vi "niScope Multi Read Cluster.vi"(7 "timeout":dbl=5.0 format="%.2f", 8 "error in":errorcluster, 9 "numSamples":i32=-1, 10 "channels":string="0", 11 "instrument handle":refnum<k15>) -> (0 "error out":errorcluster, 1 "waveform":T2(array[cluster]) {"wfm" format="%.2f"; "xIncrement" format="%.2f"; "relativeInitialX" format="%.2f"}, 2 "wfm info":T1(array[cluster]) {"reserved2" format="%.2f"; "reserved1" format="%.2f"; "offset" format="%^.3e"; "gain" format="%^.3e"; "xIncrement" format="%^.3e"; "relativeInitialX" format="%^.3e"; "absoluteInitialX" format="%^.3e"}, 3 "instrument handle out":refnum<k15>)   [LabVIEW 2013]
doc: "Initiates an acquisition, waits for it to complete, and retrieves the data for multiple channels and records."
uses:
  niScope_32.dll
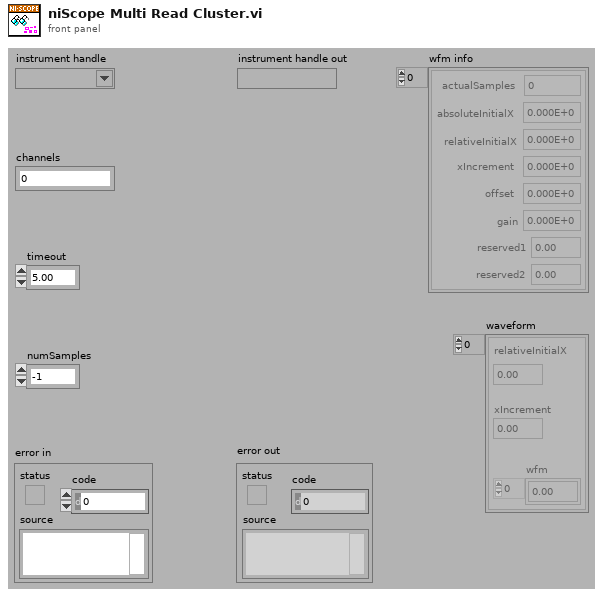
[diagram p1: front panel]
types:
  T1 = cluster{"actualSamples":i32, "absoluteInitialX":dbl, "relativeInitialX":dbl, "xIncrement":dbl, "offset":dbl, "gain":dbl, "reserved1":dbl, "reserved2":dbl}[]
  T2 = cluster{"relativeInitialX":dbl, "xIncrement":dbl, "wfm":dbl[]}[]
  T3 = cluster{"relativeInitialX":dbl, "xIncrement":dbl, "wfm":dbl[]}
  T4 = cluster{"actualSamples":i32, "absoluteInitialX":dbl, "relativeInitialX":dbl, "xIncrement":dbl, "offset":dbl, "gain":dbl, "reserved1":dbl, "reserved2":dbl}
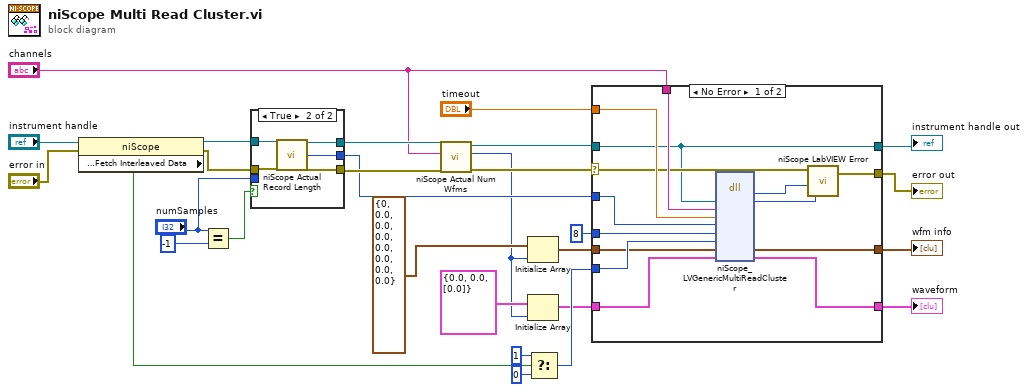
[diagram p0: block diagram]
diagram:
  n1 = property class="niScope"(reference="instrument handle", error in="error in") -> (reference out=w10:refnum<k15>, error out=w20:errorcluster, "Device Specific:IF Digitizer (5620 and 5621):Advanced:Fetch Interleaved Data"=w21:bool)
  n2 = Equal?(x="numSamples", y=-1) -> (x = y?=w27:bool)
  n3 = case shown="True" w27 {
    tunnel: [w29 w36] -> w24
    tunnel: [w30 w35] -> w25
    tunnel: "numSamples" -> [w31 _]
    tunnel: [w31 w34] -> w15
    tunnel: w10 -> [w30 w33]
    tunnel: w20 -> [w29 w32]
    frame False {
    }
    frame True {
      n4 = call <instrlib>:"niScope Actual Record Length.vi"("instrument handle"=w33, "error in"=w32) -> ("instrument handle out"=w35:refnum<k15>, "actual record length"=w34:i32, "error out"=w36:errorcluster)  [unwired: 11 in]
    }
  }
  n5 = call <instrlib>:"niScope Actual Num Wfms.vi"("error in"=w24, "channels"="channels", "instrument handle"=w25) -> ("error out"=w14:errorcluster, "actual num wfms"=w3:i32, "instrument handle out"=w13:refnum<k15>)  [unwired: 6 in]
  n6 = Initialize Array(T4 {"actualSamples"=0, "absoluteInitialX"=0.0, "relativeInitialX"=0.0, "xIncrement"=0.0, "offset"=0.0, "gain"=0.0, "reserved1"=0.0, "reserved2"=0.0} ("wfm info"), w3) -> (w2:T1)
  n7 = Initialize Array(T3 {"relativeInitialX"=0.0, "xIncrement"=0.0, "wfm"=[0.0]}, w3) -> (w1:T2)
  n8 = Select(t=1, s=w21, f=0) -> (s? t:f=w16:i32)
  n9 = case shown="No Error" w14 {
    selector: w14 -> [w38 w53]
    tunnel: [w48 w53] -> w6
    tunnel: w13 -> [w37 w54]
    tunnel: [w37 w54] -> w9
    tunnel: w15 -> [w39 _]
    tunnel: [w45 w51] -> w8
    tunnel: w16 -> [w44 _]
    tunnel: [w46 w52] -> w7
    tunnel: w1 -> [w47 w52]
    tunnel: w2 -> [w43 w51]
    tunnel: 8 ("dataType") -> [w42 _]
    tunnel: "timeout" -> [w41 _]
    tunnel: "channels" -> [w40 _]
    frame No Error {
      n10 = dll-call lib="niScope_*.*" fn="niScope_LVGenericMultiReadCluster"("instrument handle"=w37, "channel"=w40, "timeout"=w41, "numSamples"=w39, "dataType"=w42, "interleaved"=w44, "wfm_info"=w43, "in_cluster"=w47) -> ("status"=w50:i32, "instrument handle"=w49:u32, "wfm_info"=w45:T1, "in_cluster"=w46:T2)  [unwired: 8 in, 2 out]
      n11 = call <instrlib>:"niScope LabVIEW Error.vi"("instrument handle"=w49, "niScope error code (0)"=w50, "error in (no error)"=w38) -> ("error out"=w48:errorcluster)  [unwired: 2 in]
    }
    frame Error {
    }
  }
  "instrument handle out" <- w9
  "error out" <- w6
  "waveform" <- w7
  "wfm info" <- w8
